vi "Relay_Module.vi"(8 "error in":errorcluster, 10 "DUT":string) -> (0 "error in (out)":errorcluster)   [LabVIEW 2024, in "Relay_Module.lvlib"]
doc: "This template is for the Queued Message Handler design pattern.\n\nThe Event Handling Loop generates messages based on user interface actions.\n\nThe Message Handling Loop processes messages generated by the Event Handling Loop, or by other messages. The messages are string values, so new messages can be added easily to the Message Cases case structure in the Message Handling Loop. Each message cluster can also provide an optional value for Message Data, which is a variant that can be converted to whatever message-specific data is required."
uses:
  Relay_Module.lvlib
  support/Relay_Channel_Write.ctl
  support/Relay_Enum_OUT.ctl
  controls/Relay_Module UI Data.ctl
  <vilib>/NI/Modbus Library/API/master/Modbus Master.lvclass
  support/Relay_enum_IN.ctl
  PrivateControls/FGV_Queue_Control.ctl
  <vilib>/NI/Modbus Library/API/Wrapper/Create TCP Master.vi
  <vilib>/Utility/error.llb/Error Cluster From Error Code.vi
  <vilib>/ErrorRing/Error Ring.xnode
  support/Message Queue/Relay_Module Message Queue.lvlib
  support/User Event - Stop/Relay_Module User Event - Stop.lvlib
  Launcher/Launcher_DTU.lvlib
  <vilib>/NI/Modbus Library/API/Wrapper/API Main.lvlib
panel:
  in  "Config":string
  in  "Relay_Channel_Write_EOL":T1={"Relay_CH_Array"=[{"On/Off"=FALSE, "OUTPUT_Relay_Channels"=enum."GND_DMM_%d_EOL"}, {"On/Off"=FALSE, "OUTPUT_Relay_Channels"=enum."CAN_H_RES_%d_EOL"}, {"On/Off"=FALSE, "OUTPUT_Relay_Channels"=enum."CAN_L_RES_%d_EOL"}, {"On/Off"=FALSE, "OUTPUT_Relay_Channels"=enum."L_IND_RES_%d_EOL"}, {"On/Off"=FALSE, "OUTPUT_Relay_Channels"=enum."R_IND_RES_%d_EOL"}, {"On/Off"=FALSE, "OUTPUT_Relay_Channels"=enum."HB_CONN_DMM_%d_EOL"}, {"On/Off"=FALSE, "OUTPUT_Relay_Channels"=enum."14V_RES_%d_EOL"}, {"On/Off"=FALSE, "OUTPUT_Relay_Channels"=enum."CAN_L_(DMM-)_%d_EOL"}, {"On/Off"=FALSE, "OUTPUT_Relay_Channels"=enum."CAN_H_%d_EOL"}, {"On/Off"=FALSE, "OUTPUT_Relay_Channels"=enum."CAN_L_%d_EOL"}, {"On/Off"=FALSE, "OUTPUT_Relay_Channels"=enum."14V_%d_EOL"}, {"On/Off"=FALSE, "OUTPUT_Relay_Channels"=enum."GND_%d_EOL"}, {"On/Off"=FALSE, "OUTPUT_Relay_Channels"=enum."HB_CONN_%d_EOL"}, {"On/Off"=FALSE, "OUTPUT_Relay_Channels"=enum."L_IND_%d_EOL"}, {"On/Off"=FALSE, "OUTPUT_Relay_Channels"=enum."R_IND_%d_EOL"}, {"On/Off"=FALSE, "OUTPUT_Relay_Channels"=enum."CYLINDER_DUT_%d_EOL"}, {"On/Off"=FALSE, "OUTPUT_Relay_Channels"=enum."CYL_PB_1_%d_EOL"}, {"On/Off"=FALSE, "OUTPUT_Relay_Channels"=enum."CYL_PB_2_%d_EOL"}, {"On/Off"=FALSE, "OUTPUT_Relay_Channels"=enum."DUT_PASS_%d_EOL"}, {"On/Off"=FALSE, "OUTPUT_Relay_Channels"=enum."DUT_FAIL_%d_EOL"}, {"On/Off"=FALSE, "OUTPUT_Relay_Channels"=enum."SPARE1_%d_EOL"}, {"On/Off"=FALSE, "OUTPUT_Relay_Channels"=enum."Tower Red_EOL"}, {"On/Off"=FALSE, "OUTPUT_Relay_Channels"=enum."Tower Amber_EOL"}, {"On/Off"=FALSE, "OUTPUT_Relay_Channels"=enum."Tower Green_EOL"}, {"On/Off"=FALSE, "OUTPUT_Relay_Channels"=enum."Tower Buzzer_EOL"}]}
  in  "data 4":bool[](array[boolean])
  in  "data 3":bool[](array[boolean])
  in  "data 2":bool[](array[boolean])
  in  "Relay_Channel_Write":T1={"Relay_CH_Array"=[{"On/Off"=FALSE, "OUTPUT_Relay_Channels"=enum."CONN_SUPPLY_%d_FCT"}, {"On/Off"=FALSE, "OUTPUT_Relay_Channels"=enum."HB_CONN_%d_FCT"}, {"On/Off"=FALSE, "OUTPUT_Relay_Channels"=enum."L_IND_CONN_%d_FCT"}, {"On/Off"=FALSE, "OUTPUT_Relay_Channels"=enum."R_IND_CONN_%d_FCT"}, {"On/Off"=FALSE, "OUTPUT_Relay_Channels"=enum."SW1_%d_FCT"}, {"On/Off"=FALSE, "OUTPUT_Relay_Channels"=enum."SW2_%d_FCT"}, {"On/Off"=FALSE, "OUTPUT_Relay_Channels"=enum."CAN_H_%d_FCT"}, {"On/Off"=FALSE, "OUTPUT_Relay_Channels"=enum."CAN_L_%d_FCT"}, {"On/Off"=FALSE, "OUTPUT_Relay_Channels"=enum."CYLINDER_ON/OFF_%d_FCT"}, {"On/Off"=FALSE, "OUTPUT_Relay_Channels"=enum."SPARE_1_%d_FCT"}, {"On/Off"=FALSE, "OUTPUT_Relay_Channels"=enum."SPARE_2_%d_FCT"}, {"On/Off"=FALSE, "OUTPUT_Relay_Channels"=enum."Tower Red"}, {"On/Off"=FALSE, "OUTPUT_Relay_Channels"=enum."Tower Amber"}, {"On/Off"=FALSE, "OUTPUT_Relay_Channels"=enum."Tower Green"}, {"On/Off"=FALSE, "OUTPUT_Relay_Channels"=enum."Tower Buzzer"}, {"On/Off"=FALSE, "OUTPUT_Relay_Channels"=enum."SLIMRELAY_DUT_%d_FCT"}]}
  out "discrete inputs":bool[](array[boolean])
  in  "Relay_Module_IP":string
  in  "data":bool[](array[boolean])
  out "queue name 2":string
  out "queue name":string
  out "Display <Replace Me>":string
  in  "DigitalWrite":bool
  in  "Digital Read":bool
  in  "Exit":bool
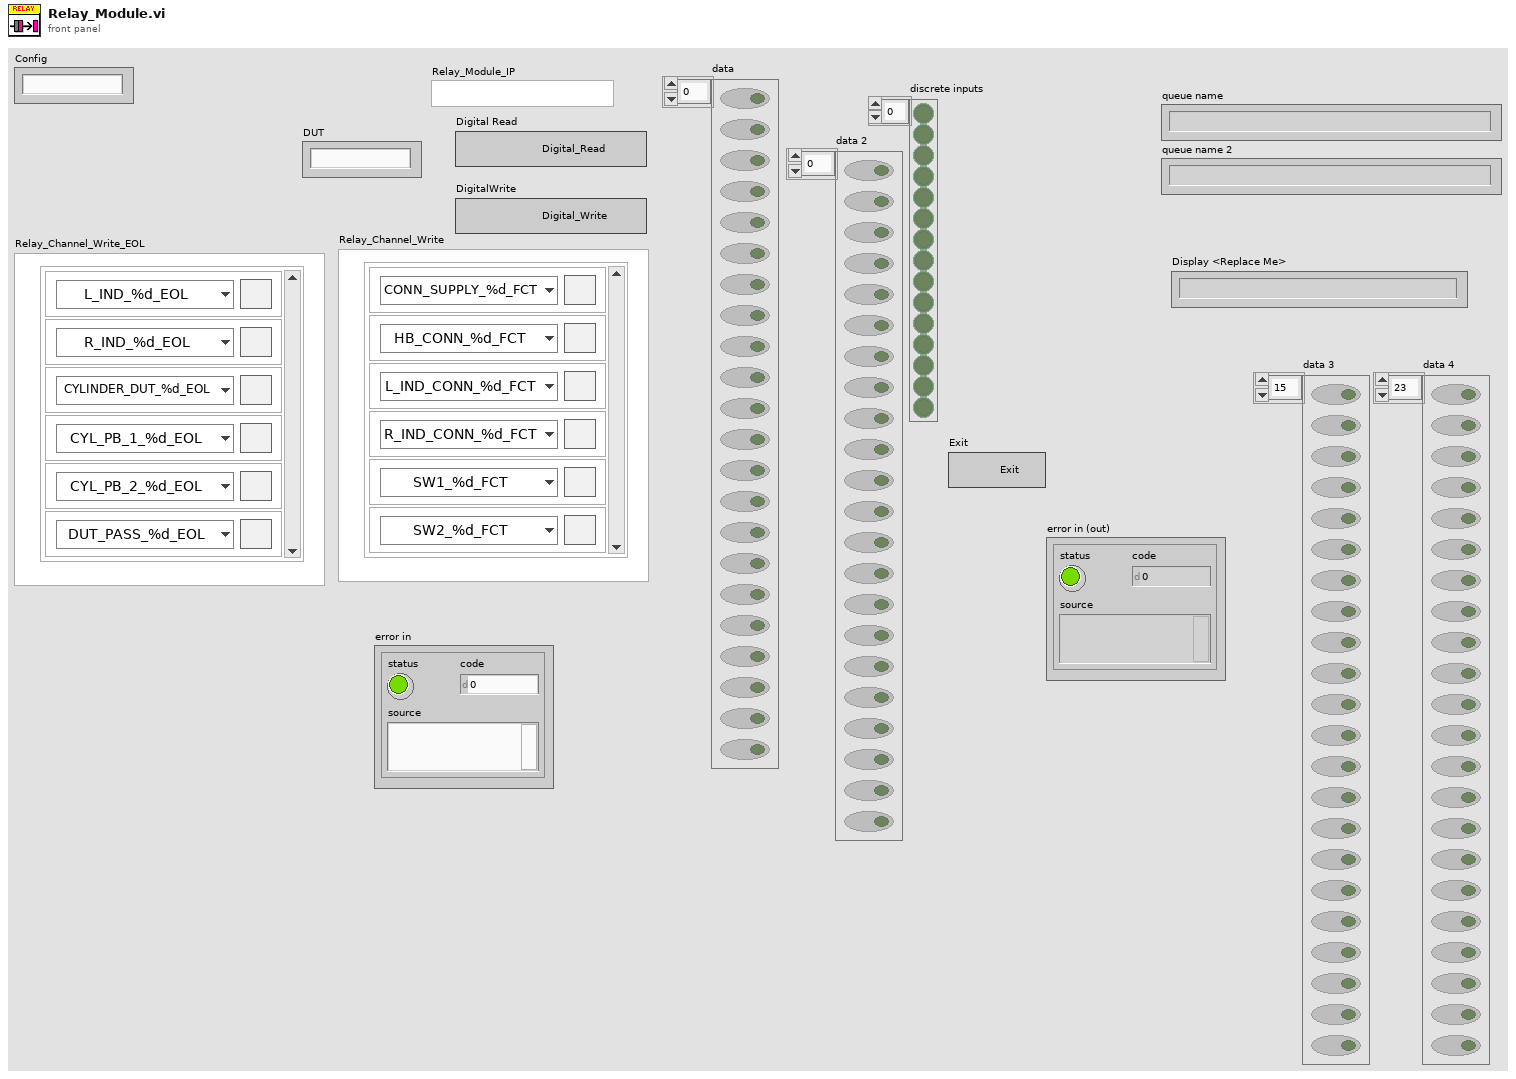
[diagram p1: front panel]
types:
  T1 = typedef "Relay_Module.lvlib/Relay_Channel_Write.ctl" = cluster{"Relay_CH_Array":cluster{"On/Off":bool, "OUTPUT_Relay_Channels":T2}[]}
  T2 = typedef "Relay_Module.lvlib/Relay_Enum_OUT.ctl" = enum16{"CONN_SUPPLY_%d_FCT", "HB_CONN_%d_FCT", "L_IND_CONN_%d_FCT", "R_IND_CONN_%d_FCT", "SW1_%d_FCT", "SW2_%d_FCT", "CAN_H_%d_FCT", "CAN_L_%d_FCT", "CYLINDER_ON/OFF_%d_FCT", "SPARE_1_%d_FCT", "SPARE_2_%d_FCT", "Tower Red", "Tower Amber", "Tower Green", "Tower Buzzer", "SLIMRELAY_DUT_%d_FCT", "GND_DMM_%d_EOL", "CAN_H_RES_%d_EOL", "CAN_L_RES_%d_EOL", "L_IND_RES_%d_EOL", "R_IND_RES_%d_EOL", "HB_CONN_DMM_%d_EOL", "14V_RES_%d_EOL", "CAN_L_(DMM-)_%d_EOL", "CAN_H_%d_EOL", "CAN_L_%d_EOL", "14V_%d_EOL", "GND_%d_EOL", "HB_CONN_%d_EOL", "L_IND_%d_EOL", "R_IND_%d_EOL", "CYLINDER_DUT_%d_EOL", "CYL_PB_1_%d_EOL", "CYL_PB_2_%d_EOL", "DUT_PASS_%d_EOL", "DUT_FAIL_%d_EOL", "SPARE1_%d_EOL", "Tower Red_EOL", "Tower Amber_EOL", "Tower Green_EOL", "Tower Buzzer_EOL"}
  T3 = typedef "Relay_Module.lvlib/Relay_Module UI Data.ctl" = cluster{"Config_Path":path, "Task_String[]":string[], "Line_String[]":string[], "DUT1_String[]":string[], "DUT2_String[]":string[], "DO_task out1":refnum<k21>, "DO_task out2":refnum<k21>, "DUT":i32, "Relay_Channel_Write":T1, "notifier out":refnum<notifier>, "serial master instance":refnum<class "Modbus Master.lvclass">, "queue In":refnum<queue>, "Config":string}
  T4 = typedef "Relay_Module.lvlib/FGV_Queue_Control.ctl" = enum16{"Release", "Get", "Set"}
  T5 = typedef "Relay_Module.lvlib/Relay_Module Message Queue.lvlib/All Message Queues.ctl" = cluster{"UI":refnum<queue>, "QSM":refnum<queue>}
  T6 = enum16{"Read", "Write", "All_sections", "All_values", "Remove key&section"}
  T7 = cluster{"Message":string, "Message Data":variant}
  T8 = typedef "Relay_Module.lvlib/Relay_enum_IN.ctl" = enum16{"EMERGENCY", "CONTROL ON", "START DUT 1", "STOP DUT 1", "PCBA PRESENCE DUT 1", "PCBA PRESENCE DUT 2", "START DUT 2", "STOP DUT 2", "EOL PRESENCE DUT 1", "EOL PRESENCE DUT 2", "LIGHT CURTAIN"}
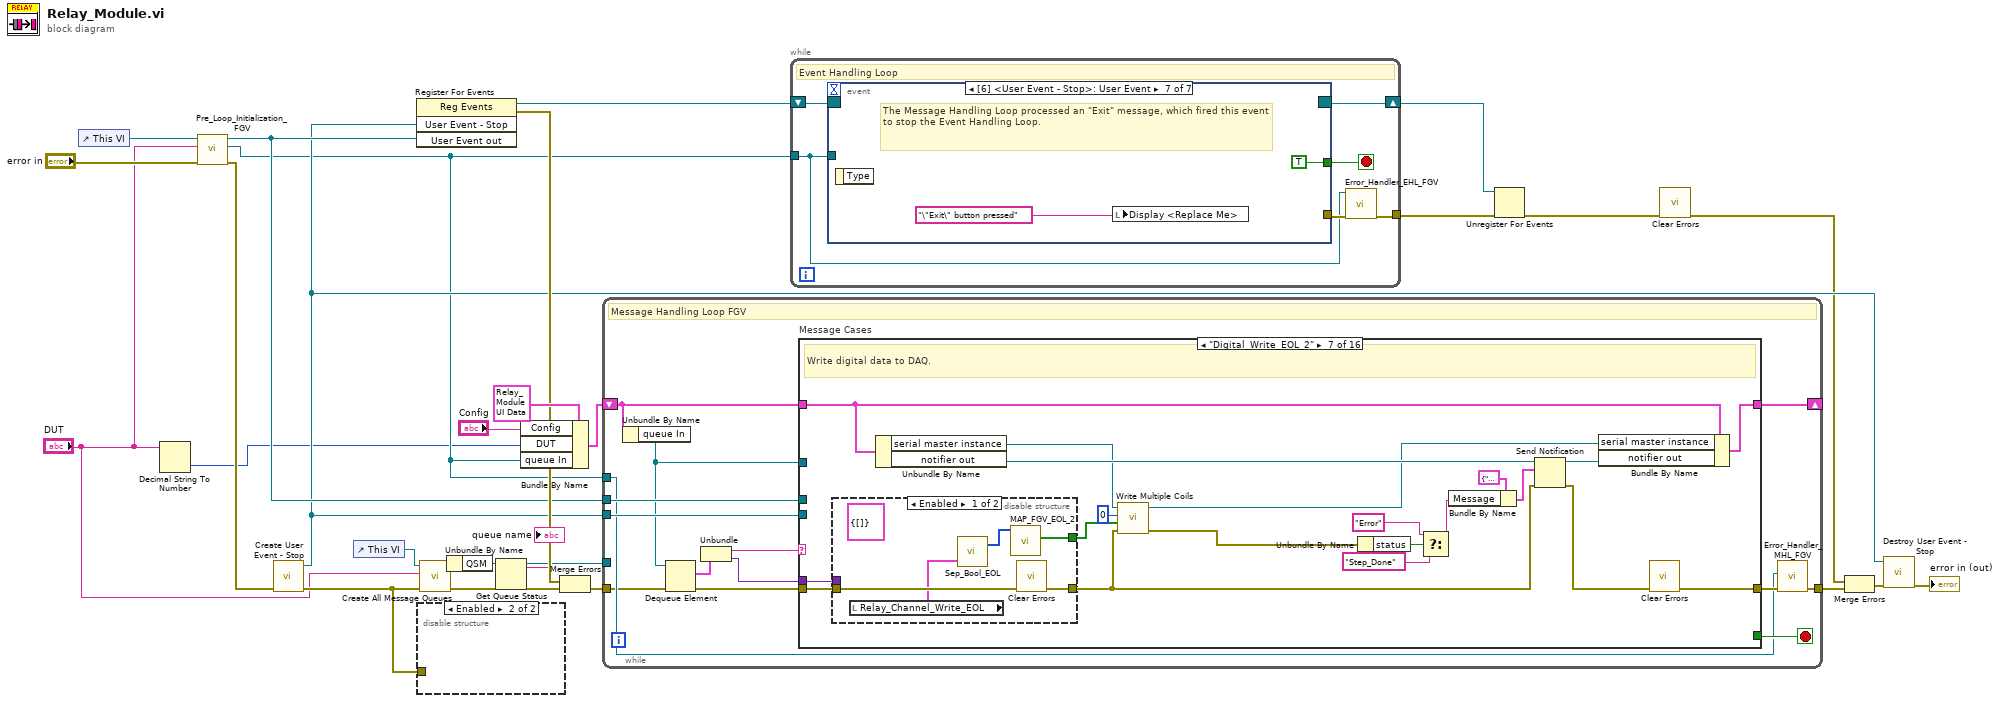
[diagram p0: block diagram]
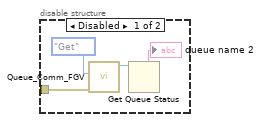
[diagram p2: hidden frame]
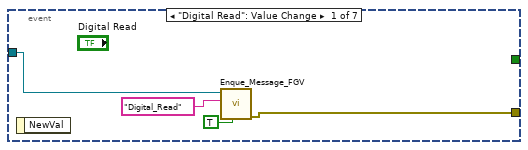
[diagram p3: hidden frame]
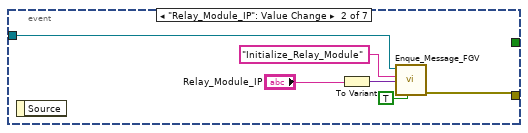
[diagram p4: hidden frame]
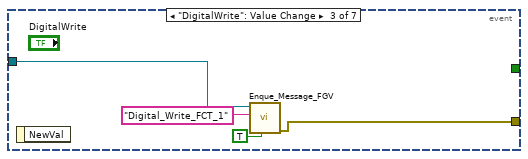
[diagram p5: hidden frame]
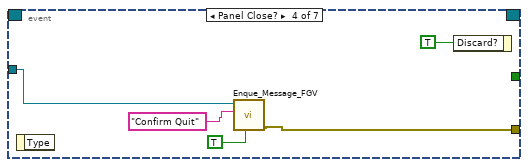
[diagram p6: hidden frame]
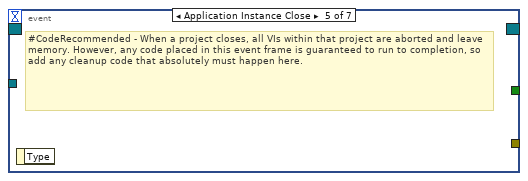
[diagram p7: hidden frame]
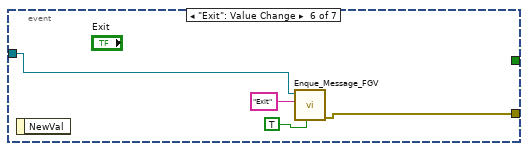
[diagram p8: hidden frame]
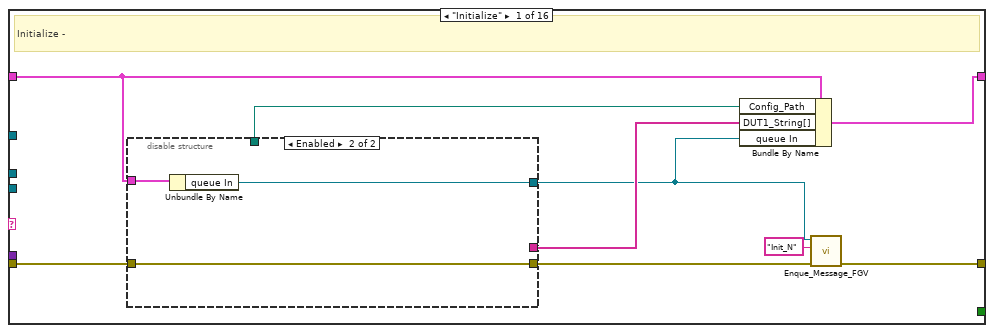
[diagram p9: hidden frame]
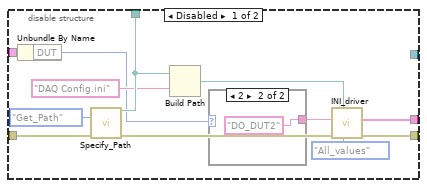
[diagram p10: hidden frame]
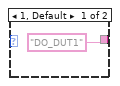
[diagram p11: hidden frame]
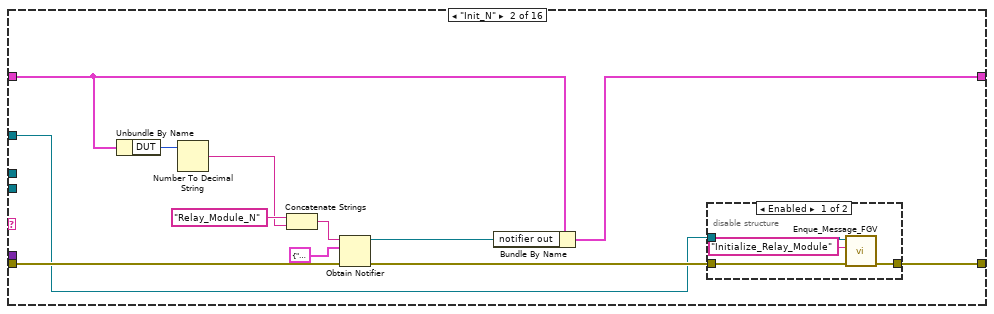
[diagram p12: hidden frame]
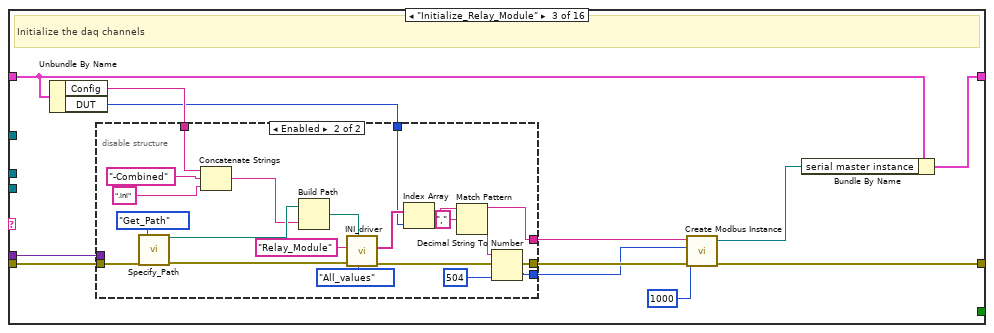
[diagram p14: hidden frame]
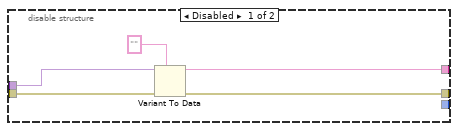
[diagram p15: hidden frame]
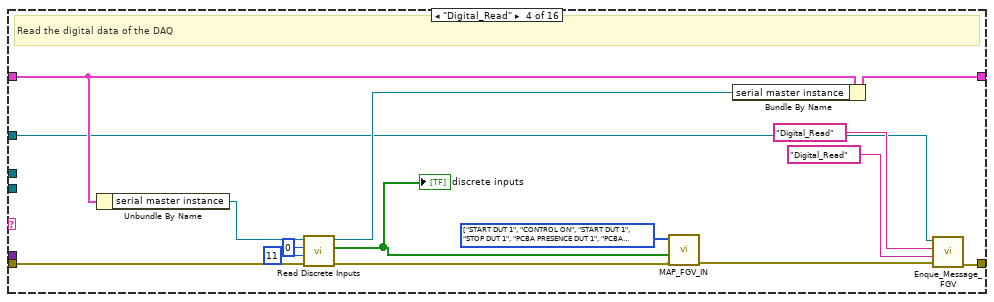
[diagram p16: hidden frame]
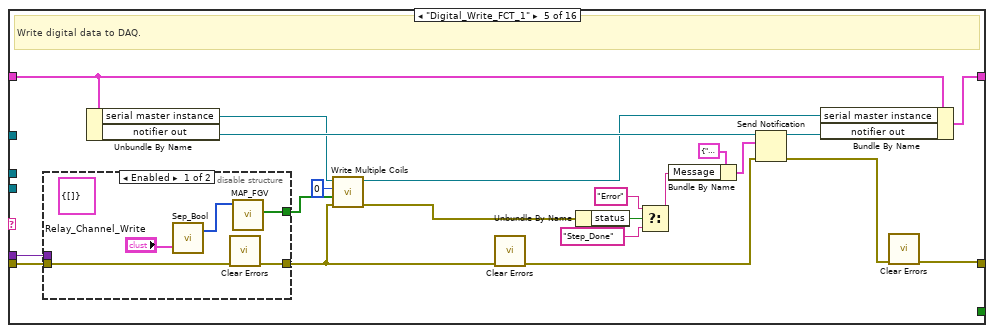
[diagram p17: hidden frame]
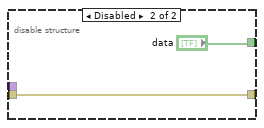
[diagram p18: hidden frame]
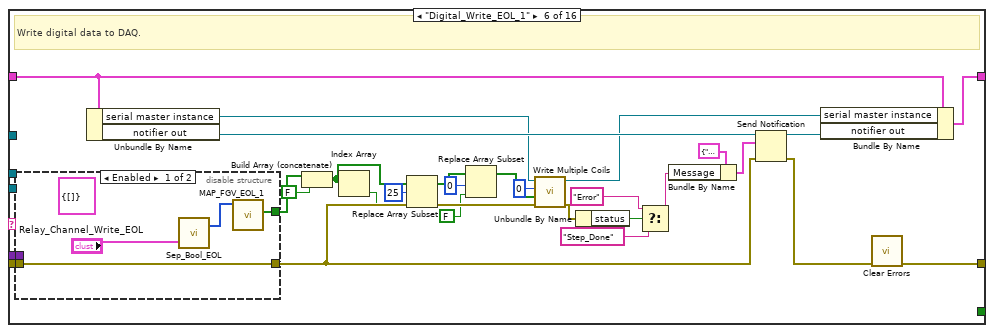
[diagram p19: hidden frame]
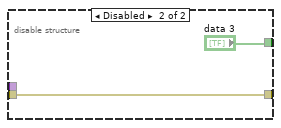
[diagram p20: hidden frame]
diagram:
  n1 = control-ref of="This VI"() -> (w16:refnum<vi>)
  n2 = Decimal String To Number(string="DUT") -> (number=w1:i32)  [unwired: 2 in, 1 out]
  n3 = call "Pre_Loop_Initialization_FGV.vi"("error in (no error)"="error in", "DUT"="DUT", "VI in"=w16) -> ("error out"=w14:errorcluster, "queue Out"=w5:refnum<queue>, "User Event out"=w8:refnum<user-event>)  [unwired: 6 in]
  n4 = call "Create User Event - Stop.vi"("error in (no error)"=w14) -> ("error out"=w9:errorcluster, "User Event - Stop"=w7:refnum<user-event>)  [unwired: 9 in]
  n5 = control-ref of="This VI"() -> (w12:refnum<vi>)
  n6 = register-events(w7, w8) -> (reference out=w19:refnum<event-registration>, error out=w17:errorcluster)  [unwired: 2 in]
  n7 = disable-structure shown="Enabled" {
    disable-tunnel: w9 -> [w32 _]
    frame Disabled {
      n8 = call "Queue_Comm_FGV.vi"("error in (no error)"=w32, "Enum"=FGV_Queue_Control."Get") -> ("queue Out"=w30:refnum<queue>)  [unwired: 8 in, 1 out]
      n9 = Get Queue Status(queue=w30) -> (queue name=→"queue name 2":string)  [unwired: 2 in, 7 out]
    }
    frame Enabled {
    }
  }
  n10 = call "Create All Message Queues.vi"("error in (no error)"=w9, "DUT"="DUT", "This VI"=w12) -> ("error out"=w28:errorcluster, "Message Queues out"=w27:T5)  [unwired: 7 in]
  n11 = Unbundle By Name(w27) -> ("QSM"=w25:refnum<queue>)
  n12 = Get Queue Status(queue=w25) -> (queue out=w11:refnum<queue>, queue name=→"queue name":string)  [unwired: 2 in, 6 out]
  n13 = Bundle By Name(cluster=T3 {"Config_Path"=path "", "Task_String[]"=[], "Line_String[]"=[], "DUT1_String[]"=[], "DUT2_String[]"=[], "DO_task out1"="", "DO_task out2"="", "DUT"=0, "Relay_Channel_Write"={"Relay_CH_Array"=[]}, "notifier out"=refnum, "serial master instance"=refnum, "queue In"=refnum, "Config"=""} ("Data Cluster"), "Config"="Config", "DUT"=w1, "queue In"=w5) -> (w6:T3)
  n14 = Merge Errors(w17, w28) -> (w18:errorcluster)
  n15 = while {
    tunnel: w11 -> [_]
    shift-right: [w46] -> _
    shift-left: w6 -> [w39]
    tunnel: w8 -> [w44]
    tunnel: w18 -> [w38]
    tunnel: [w42] -> w26
    tunnel: w7 -> [w41]
    tunnel: w5 -> [w40]
    stop <- w45 stop-if-true
    # "Message Handling Loop FGV"
    n16 = Unbundle By Name(w39) -> ("queue In"=w36:refnum<queue>)
    n17 = Dequeue Element(queue=w36, error in (no error)=w38) -> (element=w35:T7, error out=w37:errorcluster)  [unwired: 1 in, 2 out]
    n18 = Unbundle(w35) -> ("Message"=w34:string, "Message Data"=w33:variant)
    n19 = case "Message Cases" shown="\"Digital_Write_EOL_1\"" w34 {
      selector: w34 -> [_ _ _ _ _ _ _ _ _ _ _ _ _ _ _ w326]
      tunnel: w37 -> [w54 w84 w100 w137 w161 w196 w222 w249 w270 w284 w290 w300 w302 w307 w316 _]
      tunnel: [w55 w77 w101 w139 w143 w179 w204 w231 w268 w282 w291 w294 w302 w309 w311 w327] -> w43
      tunnel: w39 -> [w49 w83 w93 w138 w162 w197 w223 w250 w271 w285 w292 w299 w301 w304 w317 w328]
      tunnel: [w52 w80 w96 w133 w160 w195 w221 w248 w269 w283 w292 w299 w301 w304 w317 w328] -> w46
      tunnel: [_ _ _ _ _ _ _ _ _ _ _ _ _ _ TRUE _] -> w45
      tunnel: w33 -> [_ _ w98 _ w159 w194 w220 w247 _ _ w289 w298 _ _ _ _]
      tunnel: w44 -> [_ _ _ _ _ _ _ _ _ _ _ _ _ _ w323 _]
      tunnel: w41 -> [_ _ _ _ _ _ _ _ _ _ _ _ _ _ w320 _]
      tunnel: w36 -> [_ w73 _ w127 _ _ _ _ _ _ _ _ _ _ _ _]
      frame "Initialize" {
        # "Initialize -"
        n20 = disable-structure shown="Enabled" {
          disable-tunnel: w54 -> [w67 w72]
          disable-tunnel: [w64 w72] -> w51
          disable-tunnel: [w63 _] -> w50
          disable-tunnel: w49 -> [w59 w71]
          disable-tunnel: [w57 _] -> w48
          disable-tunnel: [_ w70] -> w47
          frame Disabled {
            n21 = Unbundle By Name(w59) -> ("DUT"=w56:i32)
            n22 = call "Specify_Path.vi"("Path_Enum"=enum16{"Find_Path", "Get_Path"}."Get_Path", "error in (no error)"=w67) -> ("Configurations"=w63:path, "error out"=w66:errorcluster)  [unwired: 6 in, 6 out]
            n23 = Build Path(base path=w63, name or relative path="DAQ Config.ini") -> (appended path=w61:path)
            n24 = case shown="2" w56 {
              tunnel: ["DO_DUT1" ("String") "DO_DUT2" ("String")] -> w58
              frame 1, Default {
              }
              frame 2 {
              }
            }
            n25 = call "INI_driver.vi"("Enum"=T6."All_values", "instrument file path"=w61, "error in (no error)"=w66, "Section"=w58) -> ("error out"=w64:errorcluster, "Values out"=w57:string[])  [unwired: 4 in, 2 out]
          }
          frame Enabled {
            n26 = Unbundle By Name(w71) -> ("queue In"=w70:refnum<queue>)
          }
        }
        n27 = Bundle By Name(cluster=w49, "Config_Path"=w50, "DUT1_String[]"=w48, "queue In"=w47) -> (w52:T3)
        n28 = call "Enque_Message_FGV.vi"("error in (no error)"=w51, "Message"="Init_N", "queue IN"=w47) -> ("error out"=w55:errorcluster)  [unwired: 8 in]
      }
      frame "Init_N" {
        n29 = Unbundle By Name(w83) -> ("DUT"=w76:i32)
        n30 = Number To Decimal String(number=w76) -> (decimal integer string=w74:string)  [unwired: 1 in]
        n31 = Concatenate Strings("Relay_Module_N" ("String"), w74) -> (w75:string)
        n32 = Obtain Notifier(name (unnamed)=w75, notification data type=T7 {"Message"="", "Message Data"=variant} ("notification"), error in (no error)=w84) -> (notifier out=w79:refnum<notifier>, error out=w78:errorcluster)  [unwired: 1 in, 1 out]
        n33 = Bundle By Name(cluster=w83, "notifier out"=w79) -> (w80:T3)
        n34 = disable-structure shown="Enabled" {
          disable-tunnel: w78 -> [w87 w89]
          disable-tunnel: [w86 w89] -> w77
          disable-tunnel: w73 -> [w85 _]
          frame Enabled {
            n35 = call "Enque_Message_FGV.vi"("error in (no error)"=w87, "Message"="Initialize_Relay_Module", "queue IN"=w85) -> ("error out"=w86:errorcluster)  [unwired: 8 in]
          }
          frame Disabled {
          }
        }
      }
      frame "Initialize_Relay_Module" {
        # "Initialize the daq channels"
        n36 = Unbundle By Name(w93) -> ("Config"=w92:string, "DUT"=w90:i32)
        n37 = disable-structure shown="Enabled" {
          disable-tunnel: w100 -> [w106 w119]
          disable-tunnel: [w105 w118] -> w99
          disable-tunnel: w98 -> [w104 _]
          disable-tunnel: [w103 w111] -> w97
          disable-tunnel: w92 -> [_ w114]
          disable-tunnel: [_ w109] -> w91
          disable-tunnel: w90 -> [_ w107]
          frame Disabled {
            n38 = Variant To Data(error in=w106, type="" ("Relay_Module_IP"), Variant=w104) -> (data=w103:string, error out=w105:errorcluster)
          }
          frame Enabled {
            n39 = call "Specify_Path.vi"("Path_Enum"=enum16{"Find_Path", "Get_Path"}."Get_Path", "error in (no error)"=w119) -> ("Configurations"=w125:path, "error out"=w122:errorcluster)  [unwired: 6 in, 6 out]
            n40 = Concatenate Strings(w114, "-Combined" ("string"), ".ini" ("string")) -> (w115:string)
            n41 = Build Path(base path=w125, name or relative path=w115) -> (appended path=w124:path)
            n42 = call "INI_driver.vi"("Enum"=T6."All_values", "instrument file path"=w124, "error in (no error)"=w122, "Section"="Relay_Module") -> ("error out"=w118:errorcluster, "Values out"=w120:string[])  [unwired: 4 in, 2 out]
            n43 = Index Array(array=w120, index=w107) -> (element=w113:string)
            n44 = Match Pattern(string=w113, regular expression=",") -> (before substring=w111:string, after substring=w110:string)  [unwired: 1 in, 2 out]
            n45 = Decimal String To Number(string=w110, default (0L)=u16 504 ("port (502)")) -> (number=w109:u16)  [unwired: 1 in, 1 out]
          }
        }
        n46 = call-poly <vilib>:"Create Modbus Instance.vi"("error in"=w99, "connect timeout ms"=1000, "port (502)"=w91, "address"=w97) -> ("error out"=w101:errorcluster, "TCP master instance"=w95:refnum<class "Modbus Master.lvclass">)  [unwired: 6 in]
        n47 = Bundle By Name(cluster=w93, "serial master instance"=w95) -> (w96:T3)
      }
      frame "Digital_Read" {
        w131 = T8[] [enum."START DUT 1", enum."CONTROL ON", enum."START DUT 1", enum."STOP DUT 1", enum."PCBA PRESENCE DUT 1", enum."PCBA PRESENCE DUT 2", enum."START DUT 2", enum."STOP DUT 2", enum."EOL PRESENCE DUT 1", enum."EOL PRESENCE DUT 2", enum."LIGHT CURTAIN"] items=["EMERGENCY", "CONTROL ON", "START DUT 1", "STOP DUT 1", "PCBA PRESENCE DUT 1", "PCBA PRESENCE DUT 2", "START DUT 2", "STOP DUT 2", "EOL PRESENCE DUT 1", "EOL PRESENCE DUT 2", "LIGHT CURTAIN"] ("PLC_BOOL_IN")
        # "Read the digital data of the DAQ"
        n48 = Unbundle By Name(w138) -> ("serial master instance"=w136:refnum<class "Modbus Master.lvclass">)
        n49 = call-dynamic "Read Discrete Inputs.vi"("error in"=w137, "number of inputs"=u16 11, "starting address"=u16 0, "Modbus master in"=w136) -> ("error out"=w130:errorcluster, "discrete inputs"=w128:bool[], "Modbus master out"=w132:refnum<class "Modbus Master.lvclass">)  [unwired: 5 in]
        "discrete inputs" <- w128
        n50 = call "MAP_FGV_IN.vi"("error in (no error)"=w130, "DOs"=w128, "Relay_ENUM_IN"=w131) -> ("error out"=w129:errorcluster)  [unwired: 6 in, 2 out]
        n51 = Bundle By Name(cluster=w138, "serial master instance"=w132) -> (w133:T3)
        n52 = call "Enque_Message_FGV.vi"("error in (no error)"=w129, "Message Data"="Digital_Read" ("\"Do Something\" button pressed"), "Message"="Digital_Read", "queue IN"=w127) -> ("error out"=w139:errorcluster)  [unwired: 7 in]
      }
      frame "Digital_Write_FCT_1" {
        # "Write digital data to DAQ."
        n53 = disable-structure shown="Enabled" {
          disable-tunnel: w161 -> [w167 w169]
          disable-tunnel: w159 -> [_ _]
          disable-tunnel: [w165 w169] -> w150
          disable-tunnel: [w164 "data"] -> w144
          frame Enabled {
            (unwired) T1 {"Relay_CH_Array"=[]} ("DAQ_Write")
            n54 = call "Sep_Bool.vi"("output cluster"="Relay_Channel_Write") -> ("Array"=w166:T2[])  [unwired: 1 in, 1 out]
            n55 = call <vilib>:"Clear Errors.vi"("error in (no error)"=w167) -> ("error out"=w165:errorcluster)  [unwired: 5 in, 1 out]
            n56 = call "MAP_FGV.vi"("Relay_Channel_Out"=w166) -> ("DOs_out"=w164:bool[])  [unwired: 8 in, 2 out]
          }
          frame Disabled {
          }
        }
        n57 = Unbundle By Name(w162) -> ("serial master instance"=w147:refnum<class "Modbus Master.lvclass">, "notifier out"=w158:refnum<notifier>)
        n58 = call-dynamic "Write Multiple Coils.vi"("error in"=w150, "coils to write"=w144, "starting address"=u16 0, "Modbus master in"=w147) -> ("error out"=w148:errorcluster, "Modbus master out"=w146:refnum<class "Modbus Master.lvclass">)  [unwired: 6 in]
        n59 = call <vilib>:"Clear Errors.vi"("error in (no error)"=w150) -> ("error out"=w142:errorcluster)  [unwired: 5 in, 1 out]
        n60 = Unbundle By Name(w148) -> ("status"=w156:bool)
        n61 = Select(t="Error", s=w156, f="Step_Done") -> (s? t:f=w154:string)
        n62 = Bundle By Name(cluster=T7 {"Message"="", "Message Data"=variant} ("notification"), "Message"=w154) -> (w153:T7)
        n63 = Send Notification(notification=w153, notifier=w158, error in (no error)=w142) -> (notifier out=w149:refnum<notifier>, error out=w151:errorcluster)
        n64 = Bundle By Name(cluster=w162, "serial master instance"=w146, "notifier out"=w149) -> (w160:T3)
        n65 = call <vilib>:"Clear Errors.vi"("error in (no error)"=w151) -> ("error out"=w143:errorcluster)  [unwired: 5 in, 1 out]
      }
      frame "Digital_Write_EOL_1" {
        # "Write digital data to DAQ."
        n66 = disable-structure shown="Enabled" {
          disable-tunnel: w196 -> [w201 w203]
          disable-tunnel: w194 -> [_ _]
          disable-tunnel: [w201 w203] -> w185
          disable-tunnel: [w200 "data 3"] -> w178
          frame Enabled {
            (unwired) T1 {"Relay_CH_Array"=[]} ("DAQ_Write")
            n67 = call "Sep_Bool_EOL.vi"("output cluster"="Relay_Channel_Write_EOL") -> ("Array"=w199:T2[])  [unwired: 1 in, 1 out]
            n68 = call "MAP_FGV_EOL_1.vi"("Relay_Channel_Out"=w199) -> ("DOs_out"=w200:bool[])  [unwired: 8 in, 2 out]
          }
          frame Disabled {
          }
        }
        n69 = Unbundle By Name(w197) -> ("serial master instance"=w182:refnum<class "Modbus Master.lvclass">, "notifier out"=w193:refnum<notifier>)
        n70 = Build Array (concatenate)(w178, FALSE) -> (w175:bool[])
        n71 = Index Array(array=w175) -> (element=w176:bool)  [unwired: 1 in]
        n72 = Replace Array Subset(array=w175, new element=w176, index=25) -> (w173:bool[])
        n73 = Replace Array Subset(array=w173, new element=FALSE, index=0) -> (w170:bool[])
        n74 = call-dynamic "Write Multiple Coils.vi"("error in"=w185, "coils to write"=w170, "starting address"=u16 0, "Modbus master in"=w182) -> ("error out"=w183:errorcluster, "Modbus master out"=w181:refnum<class "Modbus Master.lvclass">)  [unwired: 6 in]
        n75 = Unbundle By Name(w183) -> ("status"=w191:bool)
        n76 = Select(t="Error", s=w191, f="Step_Done") -> (s? t:f=w189:string)
        n77 = Bundle By Name(cluster=T7 {"Message"="", "Message Data"=variant} ("notification"), "Message"=w189) -> (w188:T7)
        n78 = Send Notification(notification=w188, notifier=w193, error in (no error)=w185) -> (notifier out=w184:refnum<notifier>, error out=w186:errorcluster)
        n79 = Bundle By Name(cluster=w197, "serial master instance"=w181, "notifier out"=w184) -> (w195:T3)
        n80 = call <vilib>:"Clear Errors.vi"("error in (no error)"=w186) -> ("error out"=w179:errorcluster)  [unwired: 5 in, 1 out]
      }
      frame "Digital_Write_EOL_2" {
        # "Write digital data to DAQ."
        n81 = disable-structure shown="Enabled" {
          disable-tunnel: w222 -> [w228 w230]
          disable-tunnel: w220 -> [_ _]
          disable-tunnel: [w227 w230] -> w211
          disable-tunnel: [w225 "data 4"] -> w205
          frame Enabled {
            (unwired) T1 {"Relay_CH_Array"=[]} ("DAQ_Write")
            n82 = local read "Relay_Channel_Write_EOL"() -> (w224:T1)
            n83 = call "Sep_Bool_EOL.vi"("output cluster"=w224) -> ("Array"=w226:T2[])  [unwired: 1 in, 1 out]
            n84 = call "MAP_FGV_EOL_2.vi"("Relay_Channel_Out"=w226) -> ("DOs_out"=w225:bool[])  [unwired: 8 in, 2 out]
            n85 = call <vilib>:"Clear Errors.vi"("error in (no error)"=w228) -> ("error out"=w227:errorcluster)  [unwired: 5 in, 1 out]
          }
          frame Disabled {
          }
        }
        n86 = Unbundle By Name(w223) -> ("serial master instance"=w208:refnum<class "Modbus Master.lvclass">, "notifier out"=w219:refnum<notifier>)
        n87 = call-dynamic "Write Multiple Coils.vi"("error in"=w211, "coils to write"=w205, "starting address"=u16 0, "Modbus master in"=w208) -> ("error out"=w209:errorcluster, "Modbus master out"=w207:refnum<class "Modbus Master.lvclass">)  [unwired: 6 in]
        n88 = Unbundle By Name(w209) -> ("status"=w217:bool)
        n89 = Select(t="Error", s=w217, f="Step_Done") -> (s? t:f=w215:string)
        n90 = Bundle By Name(cluster=T7 {"Message"="", "Message Data"=variant} ("notification"), "Message"=w215) -> (w214:T7)
        n91 = Send Notification(notification=w214, notifier=w219, error in (no error)=w211) -> (notifier out=w210:refnum<notifier>, error out=w212:errorcluster)
        n92 = Bundle By Name(cluster=w223, "serial master instance"=w207, "notifier out"=w210) -> (w221:T3)
        n93 = call <vilib>:"Clear Errors.vi"("error in (no error)"=w212) -> ("error out"=w204:errorcluster)  [unwired: 5 in, 1 out]
      }
      frame "Digital_Write_FCT_2" {
        # "Write digital data to DAQ."
        n94 = disable-structure shown="Enabled" {
          disable-tunnel: w249 -> [w255 w257]
          disable-tunnel: w247 -> [_ _]
          disable-tunnel: [w253 w257] -> w238
          disable-tunnel: [w252 "data 2"] -> w232
          frame Enabled {
            (unwired) T1 {"Relay_CH_Array"=[]} ("DAQ_Write")
            n95 = local read "Relay_Channel_Write"() -> (w251:T1)
            n96 = call "Sep_Bool.vi"("output cluster"=w251) -> ("Array"=w254:T2[])  [unwired: 1 in, 1 out]
            n97 = call <vilib>:"Clear Errors.vi"("error in (no error)"=w255) -> ("error out"=w253:errorcluster)  [unwired: 5 in, 1 out]
            n98 = call "MAP_FGV_2.vi"("Relay_Channel_Out"=w254) -> ("DOs_out"=w252:bool[])  [unwired: 8 in, 2 out]
          }
          frame Disabled {
          }
        }
        n99 = Unbundle By Name(w250) -> ("serial master instance"=w235:refnum<class "Modbus Master.lvclass">, "notifier out"=w246:refnum<notifier>)
        n100 = call-dynamic "Write Multiple Coils.vi"("error in"=w238, "coils to write"=w232, "starting address"=u16 0, "Modbus master in"=w235) -> ("error out"=w236:errorcluster, "Modbus master out"=w234:refnum<class "Modbus Master.lvclass">)  [unwired: 6 in]
        n101 = Unbundle By Name(w236) -> ("status"=w244:bool)
        n102 = Select(t="Error", s=w244, f="Step_Done") -> (s? t:f=w242:string)
        n103 = Bundle By Name(cluster=T7 {"Message"="", "Message Data"=variant} ("notification"), "Message"=w242) -> (w241:T7)
        n104 = Send Notification(notification=w241, notifier=w246, error in (no error)=w238) -> (notifier out=w237:refnum<notifier>, error out=w239:errorcluster)
        n105 = Bundle By Name(cluster=w250, "serial master instance"=w234, "notifier out"=w237) -> (w248:T3)
        n106 = call <vilib>:"Clear Errors.vi"("error in (no error)"=w239) -> ("error out"=w231:errorcluster)  [unwired: 5 in, 1 out]
      }
      frame "Towerlamp_FCT" {
        (unwired) T1 {"Relay_CH_Array"=[]} ("DAQ_Write")
        # "Write digital data to DAQ."
        n107 = local read "Relay_Channel_Write"() -> (w260:T1)
        n108 = Unbundle By Name(w271) -> ("serial master instance"=w265:refnum<class "Modbus Master.lvclass">, "notifier out"=w267:refnum<notifier>)
        n109 = call "Sep_Bool.vi"("Relay_Channel_Write"=w260) -> ("Array"=w261:T2[])  [unwired: 1 in, 1 out]
        n110 = call <vilib>:"Clear Errors.vi"("error in (no error)"=w270) -> ("error out"=w266:errorcluster)  [unwired: 5 in, 1 out]
        n111 = call "MAP_FGV.vi"("Relay_Channel_Out"=w261) -> ("DOs_out"=w262:bool[])  [unwired: 8 in, 2 out]
        n112 = call-dynamic "Write Multiple Coils.vi"("error in"=w266, "coils to write"=w262, "starting address"=u16 0, "Modbus master in"=w265) -> ("error out"=w259:errorcluster, "Modbus master out"=w264:refnum<class "Modbus Master.lvclass">)  [unwired: 6 in]
        n113 = call <vilib>:"Clear Errors.vi"("error in (no error)"=w259) -> ("error out"=w258:errorcluster)  [unwired: 5 in, 1 out]
        n114 = Merge Errors(w258) -> (w268:errorcluster)
        n115 = Bundle By Name(cluster=w271, "serial master instance"=w264, "notifier out"=w267) -> (w269:T3)
      }
      frame "Towerlamp_EOL" {
        (unwired) T1 {"Relay_CH_Array"=[]} ("DAQ_Write")
        # "Write digital data to DAQ."
        n116 = local read "Relay_Channel_Write_EOL"() -> (w273:T1)
        n117 = Unbundle By Name(w285) -> ("serial master instance"=w279:refnum<class "Modbus Master.lvclass">, "notifier out"=w281:refnum<notifier>)
        n118 = call "Sep_Bool_EOL.vi"("Relay_Channel_Write"=w273) -> ("Array"=w274:T2[])  [unwired: 1 in, 1 out]
        n119 = call <vilib>:"Clear Errors.vi"("error in (no error)"=w284) -> ("error out"=w280:errorcluster)  [unwired: 5 in, 1 out]
        n120 = call "MAP_FGV_EOL_1.vi"("Relay_Channel_Out"=w274) -> ("DOs_out"=w275:bool[])  [unwired: 8 in, 2 out]
        n121 = call-dynamic "Write Multiple Coils.vi"("error in"=w280, "coils to write"=w275, "starting address"=u16 0, "Modbus master in"=w279) -> ("error out"=w276:errorcluster, "Modbus master out"=w278:refnum<class "Modbus Master.lvclass">)  [unwired: 6 in]
        n122 = call <vilib>:"Clear Errors.vi"("error in (no error)"=w276) -> ("error out"=w272:errorcluster)  [unwired: 5 in, 1 out]
        n123 = Merge Errors(w272) -> (w282:errorcluster)
        n124 = Bundle By Name(cluster=w285, "serial master instance"=w278, "notifier out"=w281) -> (w283:T3)
      }
      frame "Update Display" {
        # "Update Display - Convert the message data to a string to display in the Data Display indicator."
        n125 = Variant To Data(error in=w290, type="", Variant=w289) -> (data=→"Display <Replace Me>":string, error out=w287:errorcluster)
        n126 = Merge Errors(w287) -> (w291:errorcluster)
      }
      frame "Error" {
        # "Error - Display an error dialog. This message is sent by the \"Error Handler\" VIs at the end of other loops in this application."
        n127 = Variant To Data(error in=w300, type=errorcluster {"status"=FALSE, "code"=0, "source"=""} ("error constant"), Variant=w298) -> (data=w296:errorcluster, error out=w295:errorcluster)
        n128 = call <vilib>:"Simple Error Handler.vi"("error in (no error)"=w296) -> ()  [unwired: 4 in, 5 out]
        n129 = call <vilib>:"Clear Errors.vi"("error in (no error)"=w295) -> ("error out"=w293:errorcluster)  [unwired: 5 in, 1 out]
        n130 = Merge Errors(w293) -> (w294:errorcluster)
      }
      frame "Reset" {
      }
      frame "Confirm Quit" {
        # "Confirm Quit - Message that can confirm whether or not the user wants to exit the application."
        n131 = Unbundle By Name(w304) -> ("queue In"=w303:refnum<queue>)
        n132 = call "Enque_Message_FGV.vi"("Priority"=TRUE ("Priority Message? (F)"), "error in (no error)"=w307, "Message"="Exit", "queue IN"=w303) -> ("error out"=w308:errorcluster)  [unwired: 7 in]
        n133 = Merge Errors(w308) -> (w309:errorcluster)
      }
      frame "Exit" {
        # "Exit - Exit the application."
        n134 = Unbundle By Name(w317) -> ("serial master instance"=w312:refnum<class "Modbus Master.lvclass">, "notifier out"=w314:refnum<notifier>, "queue In"=w310:refnum<queue>)
        n135 = call "Queue_Comm_FGV.vi"("error in (no error)"=w316, "Enum"=FGV_Queue_Control."Release", "queue in"=w310) -> ("error Out"=w321:errorcluster)  [unwired: 7 in, 1 out]
        n136 = call-dynamic "Shutdown.vi"("error in"=w316, "Modbus master in"=w312) -> ("error out"=w313:errorcluster)  [unwired: 9 in]
        n137 = Release Notifier(notifier=w314, error in (no error)=w316) -> (error out=w315:errorcluster)  [unwired: 1 in, 2 out]
        n138 = call "Fire User Event - Stop.vi"("User Event - Stop"=w320) -> ("error out"=w318:errorcluster)  [unwired: 10 in]
        n139 = call "Fire User Event - Stop.vi"("User Event - Stop"=w323) -> ("error out"=w319:errorcluster)  [unwired: 10 in]
        n140 = Merge Errors(w313, w315, w319, w318, w321) -> (w324:errorcluster)
        n141 = call <vilib>:"Clear Errors.vi"("error in (no error)"=w324) -> ("error out"=w311:errorcluster)  [unwired: 5 in, 1 out]
      }
      frame Default {
        # "'Default' case only runs if there is a message that isn't defined in any of the other cases.  Output a programming error."
        n142 = xnode "Error Ring"("parameter 0"=w326) -> ("error out"=w327:errorcluster)
      }
    }
    n143 = call "Error_Handler_MHL_FGV.vi"("error in (no error)"=w43, "queue IN"=w40) -> ("error Out"=w42:errorcluster)  [unwired: 9 in]
  }
  n144 = while {
    shift-right: [w340] -> w22
    shift-left: w19 -> [w341]
    tunnel: [w337] -> w20
    tunnel: w5 -> [w336]
    stop <- w339 stop-if-true
    # "Event Handling Loop"
    n145 = event shown="[6] <User Event - Stop>: User Event" {
      selector: w341 -> [_ _ _ _ _ _ _]
      dyn-events: [_ _ _ _ _ _ _] -> w340
      timeout: _ -> [_ _ _ _ _ _ _]
      tunnel: [_ _ _ _ _ _ TRUE ("Discard?")] -> w339
      tunnel: [w344 w349 w353 w359 _ w364 _] -> w338
      tunnel: w336 -> [w342 w346 w352 w356 _ w361 _]
      event "Digital Read": Value Change {
        n146 = event-data() -> ()  [unwired: 1 in, 1 out]
        n147 = call "Enque_Message_FGV.vi"("Priority"=TRUE ("Priority Message? (F)"), "Message"="Digital_Read", "queue IN"=w342) -> ("error out"=w344:errorcluster)  [unwired: 8 in]
      }
      event "Relay_Module_IP": Value Change {
        n148 = event-data() -> ()  [unwired: 1 in, 1 out]
        n149 = To Variant(anything="Relay_Module_IP") -> (Variant=w348:variant)
        n150 = call "Enque_Message_FGV.vi"("Priority"=TRUE ("Priority Message? (F)"), "Message Data"=w348, "Message"="Initialize_Relay_Module", "queue IN"=w346) -> ("error out"=w349:errorcluster)  [unwired: 7 in]
      }
      event "DigitalWrite": Value Change {
        n151 = event-data() -> ()  [unwired: 1 in, 1 out]
        n152 = call "Enque_Message_FGV.vi"("Priority"=TRUE ("Priority Message? (F)"), "Message"="Digital_Write_FCT_1", "queue IN"=w352) -> ("error out"=w353:errorcluster)  [unwired: 8 in]
      }
      event Panel Close? {
        n153 = event-data() -> ()  [unwired: 1 in, 1 out]
        n154 = call "Enque_Message_FGV.vi"("Priority"=TRUE ("Priority Message? (F)"), "Message"="Confirm Quit", "queue IN"=w356) -> ("error out"=w359:errorcluster)  [unwired: 8 in]
        n155 = event-data("Discard?"=TRUE) -> ()  [unwired: 1 in, 1 out]
      }
      event Application Instance Close {
        # "#CodeRecommended - When a project closes, all VIs within that project are aborted and leave memory. However, any code placed in this event frame is guaranteed to run to completion, so add any cleanup code that absolutely must happen here."
        n156 = event-data() -> ()  [unwired: 1 in, 1 out]
      }
      event "Exit": Value Change {
        n157 = event-data() -> ()  [unwired: 1 in, 1 out]
        n158 = call "Enque_Message_FGV.vi"("Priority"=TRUE ("Priority Message? (F)"), "Message"="Exit", "queue IN"=w361) -> ("error out"=w364:errorcluster)  [unwired: 8 in]
      }
      event User Event {
        # "The Message Handling Loop processed an \"Exit\" message, which fired this event to stop the Event Handling Loop."
        n159 = event-data() -> ()  [unwired: 1 in, 1 out]
        n160 = local write "Display <Replace Me>"("\"Exit\" button pressed" ("VI Stopped")) -> ()
      }
    }
    n161 = call "Error_Handler_EHL_FGV.vi"("error in (no error)"=w338, "queue IN"=w336) -> ("error Out"=w337:errorcluster)  [unwired: 9 in]
  }
  n162 = Unregister For Events(event registration refnum=w22, error in=w20) -> (error out=w23:errorcluster)
  n163 = call <vilib>:"Clear Errors.vi"("error in (no error)"=w23) -> ("error out"=w4:errorcluster)  [unwired: 5 in, 1 out]
  n164 = Merge Errors(w4, w26) -> (w24:errorcluster)
  n165 = call "Destroy User Event - Stop.vi"("error in (no error)"=w24, "User Event - Stop"=w7) -> ("error out"=→"error in (out)":errorcluster)  [unwired: 9 in]
